vi "External Actuator Data Set.vi"(7 "Selected Actuator":T2, 8 "error in (no error)":errorcluster, 9 "Volts In":T1, 10 "External Actuator Data In":T1, 11 "Measurement Actions":T3) -> (0 "error out":errorcluster, 1 "Volts Out":T1, 2 "Actuator Data Out":T1)   [LabVIEW 2009]
uses:
  Actuator Measurment Actions.ctl
  Data Access Objects/External Actuators/External Actuator Id.ctl
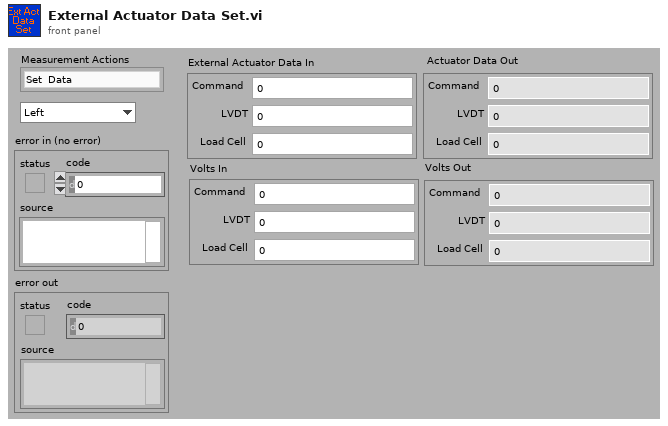
[diagram p1: front panel]
types:
  T1 = cluster{"Command":dbl, "LVDT":dbl, "Load Cell":dbl}
  T2 = typedef "External Actuator Id.ctl" = enum16{"Left", "Right"}
  T3 = typedef "Actuator Measurment Actions.ctl" = enum16{"Set  Data", "Get", "Init"}
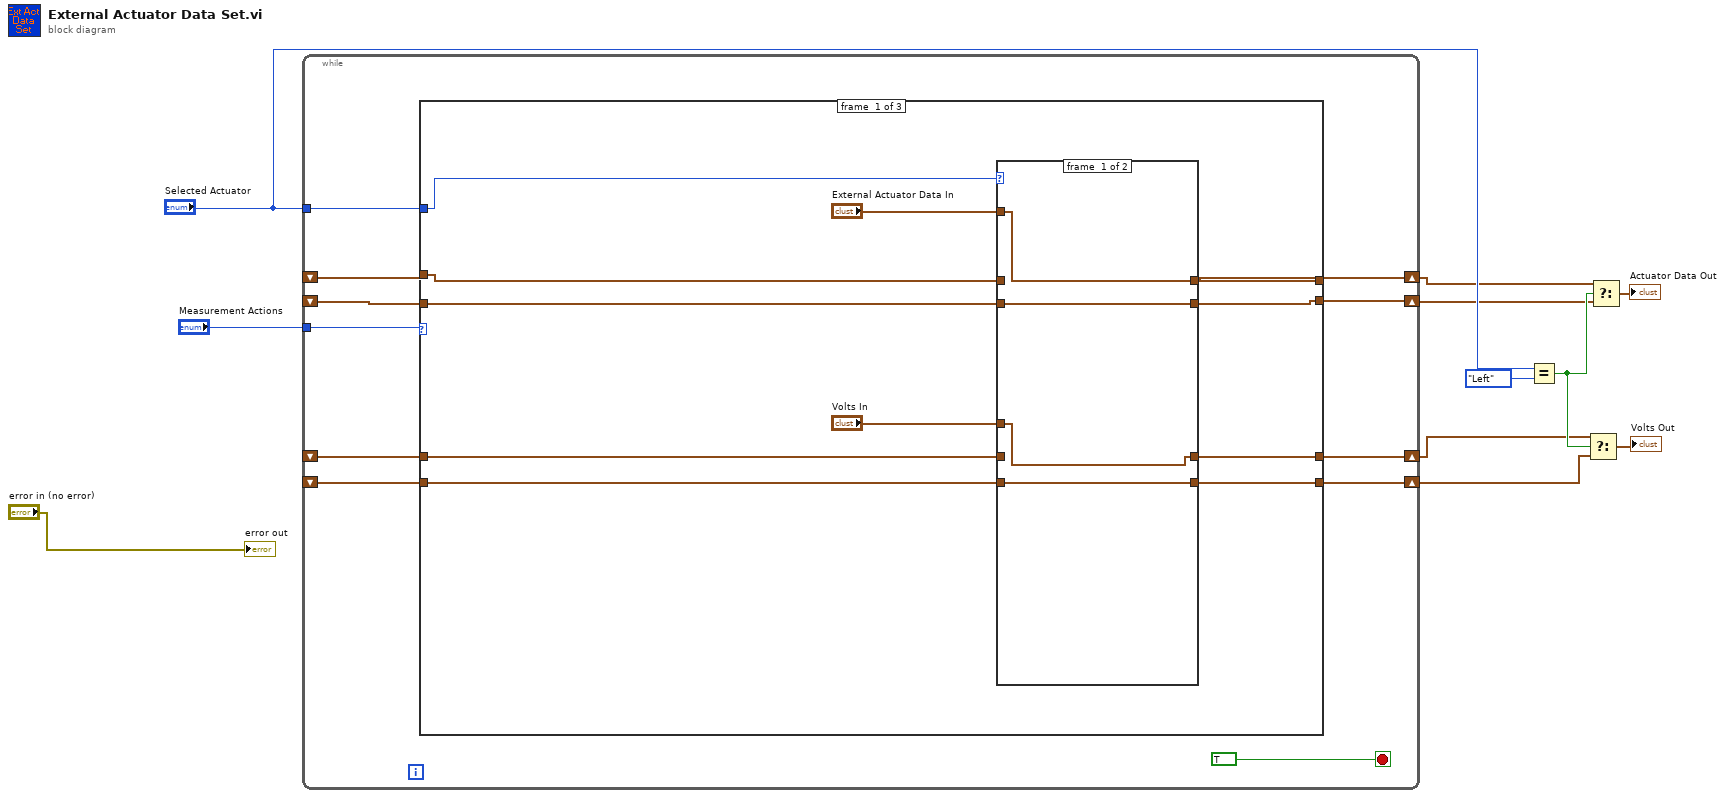
[diagram p0: block diagram]
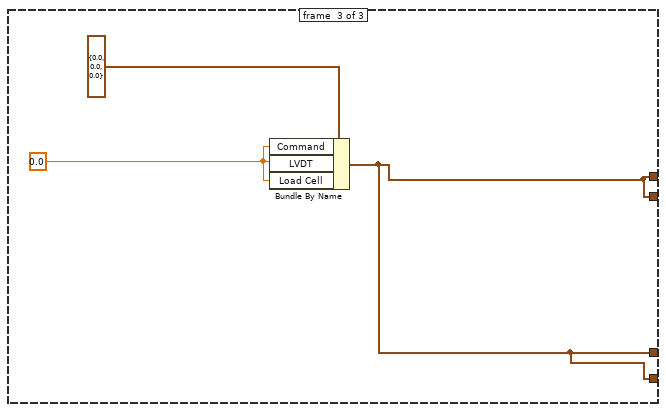
[diagram p4: hidden frame]
diagram:
  n1 = while {
    tunnel: "Measurement Actions" -> [w22]
    shift-right: [w20] -> w3
    shift-left: _ -> [w18]
    shift-right: [w19] -> w4
    shift-left: _ -> [w17]
    tunnel: "Selected Actuator" -> [w16]
    shift-right: [w15] -> w1
    shift-left: _ -> [w13]
    shift-right: [w14] -> w2
    shift-left: _ -> [w12]
    stop <- TRUE stop-if-true
    n2 = case shown="\"Init\"" w22 {
      tunnel: [w27 w45 w47] -> w20
      tunnel: [w30 w44 w47] -> w19
      tunnel: w18 -> [w28 w45 _]
      tunnel: w17 -> [w26 w44 _]
      tunnel: w16 -> [w33 _ _]
      tunnel: [w29 w42 w47] -> w15
      tunnel: [w25 w43 w47] -> w14
      tunnel: w13 -> [w24 w42 _]
      tunnel: w12 -> [w23 w43 _]
      frame #0 {
        n3 = case shown="\"Right\"" w33 {
          tunnel: "Volts In" -> [w35 w39]
          tunnel: "External Actuator Data In" -> [w37 w40]
          tunnel: [w37 w41] -> w30
          tunnel: [w34 w39] -> w29
          tunnel: w28 -> [w36 _]
          tunnel: [w36 w40] -> w27
          tunnel: w26 -> [_ w41]
          tunnel: [w35 w38] -> w25
          tunnel: w24 -> [w34 _]
          tunnel: w23 -> [_ w38]
          frame #0 {
          }
          frame #1 {
          }
        }
      }
      frame #1 {
      }
      frame #2 {
        w46 = 0.0
        n4 = Bundle By Name(cluster=T1 {"Command"=0.0, "LVDT"=0.0, "Load Cell"=0.0} ("Actuator Data Out"), "Command"=w46, "LVDT"=w46, "Load Cell"=w46) -> (w47:T1)
      }
    }
  }
  n5 = Equal?(x="Selected Actuator", y=External_Actuator_Id."Left") -> (x = y?=w7:bool)
  n6 = Select(t=w2, s=w7, f=w1) -> (s? t:f=→"Volts Out":T1)
  n7 = Select(t=w4, s=w7, f=w3) -> (s? t:f=→"Actuator Data Out":T1)
  "error out" <- "error in (no error)"
